vi "Stop Acquisition.vi"(8 "error in (no error)":errorcluster, 11 "VISA":T1) -> (0 "error out":errorcluster)   [LabVIEW 2016, in "Acquisition.lvlib"]
doc: "Stops the acquisition."
uses:
  Acquisition.lvlib
  Hardware Configuration.ctl
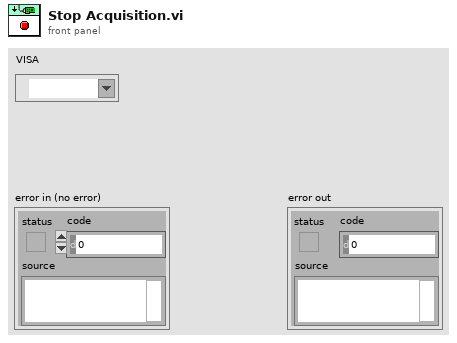
[diagram p1: front panel]
types:
  T1 = typedef "Acquisition.lvlib/Hardware Configuration.ctl" = refnum<visa-resource-name>
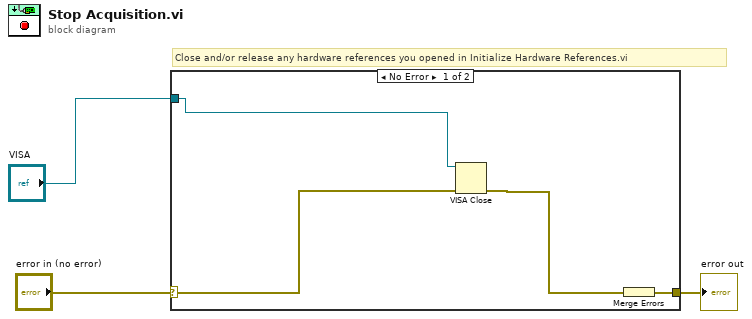
[diagram p0: block diagram]
diagram:
  # "Close and/or release any hardware references you opened in Initialize Hardware References.vi"
  n1 = case shown="No Error" "error in (no error)" {
    selector: "error in (no error)" -> [w5 w8]
    tunnel: [w7 w8] -> w2
    tunnel: "VISA" -> [w4 _]
    frame No Error {
      n2 = VISA Close(VISA resource name=w4, error in (no error)=w5) -> (error out=w6:errorcluster)
      n3 = Merge Errors(w6) -> (w7:errorcluster)
    }
    frame Error {
    }
  }
  "error out" <- w2
